vi "Get_WavelengthPower.vi"(8 "error in (no error)":errorcluster, 10 "Index":u8, 11 "NKT in":refnum<class "NKT_Extreme.lvclass">) -> (0 "error out":errorcluster, 1 "Power":dbl, 2 "Wavelength":dbl[unit], 3 "NKT out":refnum<class "NKT_Extreme.lvclass">)   [LabVIEW 2020, in "NKT_Extreme.lvclass"]
uses:
  <instrlib>/Classes/Laser/NKT/NKT_Extreme.lvclass
  <instrlib>/NKTP_API/NKTP_API.lvlib
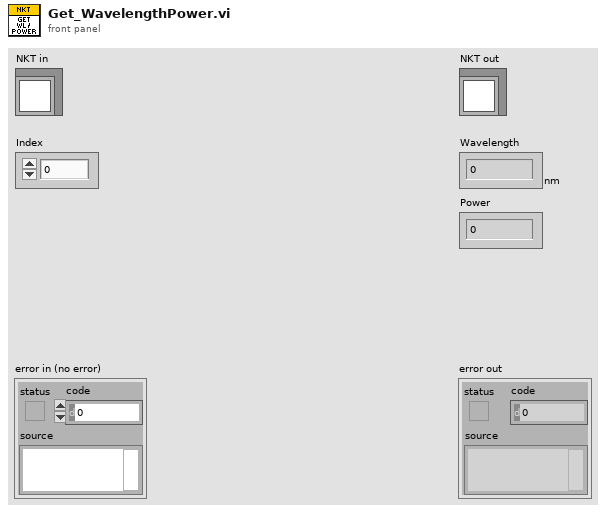
[diagram p1: front panel]
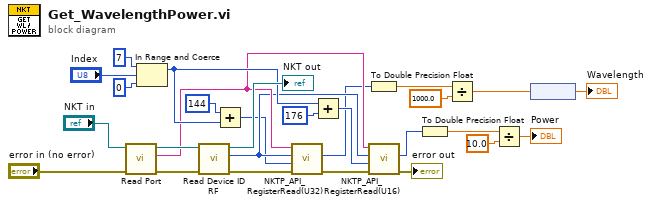
[diagram p0: block diagram]
diagram:
  n1 = call-dynamic "Read Port.vi"("error in (no error)"="error in (no error)", "NKT in"="NKT in") -> ("error out"=w24:errorcluster, "Port"=w16:string, "NKT out"=w25:refnum<class "NKT_Extreme.lvclass">)  [unwired: 7 in]
  n2 = In Range and Coerce(upper limit=u8 7, x="Index", lower limit=u8 0) -> (coerced(x)=w19:u8)  [unwired: 1 out]
  n3 = call-dynamic "Read Device ID RF.vi"("error in (no error)"=w24, "NKT in"=w25) -> ("error out"=w14:errorcluster, "Device ID RF"=w15:u8, "NKT out"=→"NKT out":refnum<class "NKT_Extreme.lvclass">)  [unwired: 7 in]
  n4 = Add(x=u8 144 ("regId"), y=w19) -> (x+y=w11:u8)
  n5 = call <instrlib>:"NKTP_API_RegisterRead(U32).vi"("error in"=w14, "regId"=w11, "devId"=w15, "portname"=w16) -> ("error out"=w13:errorcluster, "value"=w9:u32)  [unwired: 5 in, 1 out]
  n6 = Add(x=w19, y=u8 176 ("regId")) -> (x+y=w10:u8)
  n7 = To Double Precision Float(number=w9) -> (double precision float=w8:dbl)
  n8 = call <instrlib>:"NKTP_API_RegisterRead(U16).vi"("error in"=w13, "regId"=w10, "devId"=w15, "portname"=w16) -> ("error out"=→"error out":errorcluster, "value"=w4:u16)  [unwired: 5 in, 1 out]
  n9 = To Double Precision Float(number=w4) -> (double precision float=w3:dbl)
  n10 = Divide(x=w8, y=1000.0) -> (x/y=w6:dbl)
  n11 = Divide(x=w3, y=10.0) -> (x/y=→"Power":dbl)
  n12 = node(w6) -> (→"Wavelength":dbl[unit])
